vi "Begin.vi"(8 "error in":errorcluster) -> (0 "error out":errorcluster)   [LabVIEW 2020]
doc: "Called before other user functions, this VI is expected to open initial I/O refnums, load in file data, and do all program initialization. Notice that the <B>error out</B> terminal is simply used for data flow. Wiring it to other structures or subVIs ensures that this VI runs first."
uses:
  <vilib>/Rock Robotics/WPI/DriverStation/WPI_DriverStationRobotMode2.ctl
  <vilib>/Rock Robotics/WPI/ThirdParty/REV Robotics/REVLib/Typedef/Spark MAX Motor Type.ctl
  <vilib>/Rock Robotics/WPI/ThirdParty/REV Robotics/REVLib/Typedef/Spark MAX Sensor Type.ctl
  <vilib>/Rock Robotics/WPI/Joystick/WPI_JoystickDeviceEnum.ctl
  <vilib>/Rock Robotics/WPI/Solenoid/WPI_SolenoidChannel.ctl
  <vilib>/Rock Robotics/WPI/SafetyOutput/WPI_SafetyOutputConfigMenu.ctl
  <vilib>/Rock Robotics/SystemInterfaces/DIO/FPGA_DIOChannel.ctl
  Robot Global Data.vi
  <vilib>/Rock Robotics/Network Tables/NT Write String Array.vi
  <vilib>/Rock Robotics/WPI/RobotDrive/WPI_RobotDriveOpen2MotorWithExistingMotors.vi
  <vilib>/Rock Robotics/WPI/Solenoid/WPI_SolenoidOpenDouble.vi
  <vilib>/Rock Robotics/WPI/Utilities/WPI_GetSetVariantRefNum.vi
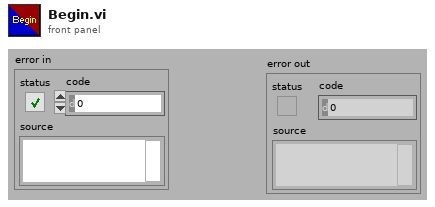
[diagram p1: front panel]
types:
  T1 = typedef "Spark MAX Sensor Type.ctl" = enum16{"No Sensor", "Hall Sensor", "Encoder", "-Not Available-", "Analog", "Alternate Encoder"}
  T2 = typedef "Spark MAX Motor Type.ctl" = enum16{"Brushed", "Brushless"}
  T3 = typedef "FPGA_DIOChannel.ctl" = enum8{"DIO 0", "DIO 1", "DIO 2", "DIO 3", "DIO 4", "DIO 5", "DIO 6", "DIO 7", "DIO 8", "DIO 9", "DIO MXP 0", "DIO MXP 1", "DIO MXP 2", "DIO MXP 3", "DIO MXP 4", "DIO MXP 5", "DIO MXP 6", "DIO MXP 7", "DIO MXP 8", "DIO MXP 9", "DIO MXP 10", "DIO MXP 11", "DIO MXP 12", "DIO MXP 13", "DIO MXP 14", "DIO MXP 15", "SPI Port CS1", "SPI Port CS2", "SPI Port CS3", "SPI Port MISO", "SPI Port MOSI", "Invalid"}
  T4 = typedef "WPI_SafetyOutputConfigMenu.ctl" = enum16{"Enable", "Disable"}
  T5 = typedef "WPI_SolenoidChannel.ctl" = enum8{"Solenoid 0", "Solenoid 1", "Solenoid 2", "Solenoid 3", "Solenoid 4", "Solenoid 5", "Solenoid 6", "Solenoid 7", "Solenoid 8", "Solenoid 9", "Solenoid 10", "Solenoid 11", "Solenoid 12", "Solenoid 13", "Solenoid 14", "Solenoid 15", "Invalid"}
  T6 = typedef "WPI_JoystickDeviceEnum.ctl" = enum16{"USB 0", "USB 1", "USB 2", "USB 3", "USB 4", "USB 5"}
  T7 = typedef "WPI_DriverStationRobotMode2.ctl" = enum16{"Autonomous Disabled", "Autonomous Enabled", "Teleop Disabled", "Teleop Enabled", "Disconnected", "Finish", "Test Disabled", "Test Enabled", "Emergency Stopped"}
  T8 = typedef "WPI_MotorControlDeviceRef.ctl" = cluster{"DeviceStatus":errorcluster, "Type":T9, "PWM":cluster{"PWM Channel":T10, "DeadBand":T11}, "CAN":cluster{"Device Number":u8, "SetOutput VI Ref":variant, "GetOutput VI Ref":variant, "Enable VI Ref":variant, "Disable VI Ref":variant, "Data":variant}, "Invert":bool, "DIO PWM":cluster{"PWM \"Enable\" Channel":T10, "DIOChannel":T3, "PWM Rate":dbl}}
  T9 = typedef "WPI_MotorControlType.ctl" = enum16{"PWM", "CAN", "DIO PWM"}
  T10 = typedef "FPGA_DIOPWMChannel.ctl" = enum8{"PWM 0", "PWM 1", "PWM 2", "PWM 3", "PWM 4", "PWM 5", "PWM 6", "PWM 7", "PWM 8", "PWM 9", "PWM MXP 0", "PWM MXP 1", "PWM MXP 2", "PWM MXP 3", "PWM MXP 4", "PWM MXP 5", "PWM MXP 6", "PWM MXP 7", "PWM MXP 8", "PWM MXP 9", "Invalid"}
  T11 = typedef "WPI_PWMDeadband.ctl" = cluster{"Name":string, "maxPositivePwm":i32, "minPositivePwm":i32, "centerPwm":i32, "maxNegativePwm":i32, "minNegativePwm":i32, "angularRange":u16}
  T12 = typedef "WPI_JoystickDevRef.ctl" = cluster{"Device":T6}
  T13 = typedef "WPI_RobotDriveDevRef.ctl" = cluster{"DevStatus":errorcluster, "Motors[]":T8[], "Square Inputs":bool, "Max Output":dbl}
  T14 = typedef "WPI_SolenoidDevRef.ctl" = cluster{"DevStatus":errorcluster, "Pneumatics Control Module":u8, "Forward Solenoid Channel":T5, "Reverse Solenoid Channel":T5}
  T15 = typedef "WPI_CompressorDevRef.ctl" = cluster{"DevStatus":errorcluster, "Pneumatics Control Module":u8}
  T16 = typedef "WPI_DigitalInputDevRef.ctl" = cluster{"DevStatus":errorcluster, "DIO Channel":T3}
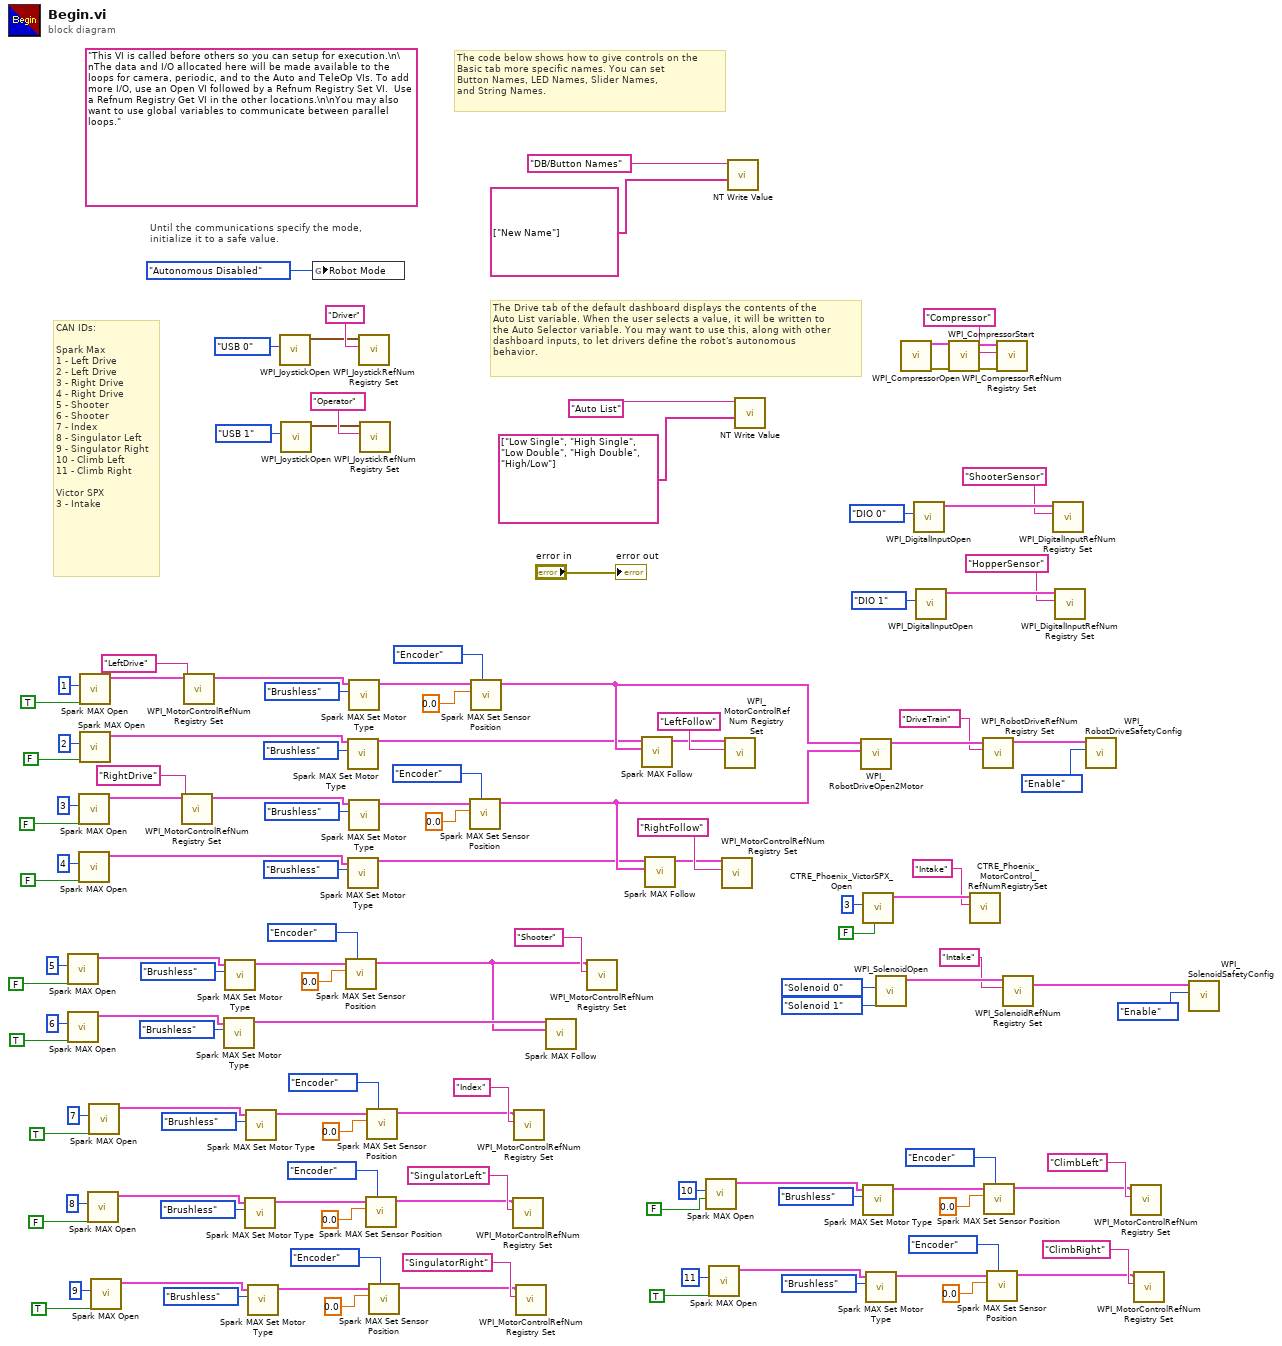
[diagram p0: block diagram]
diagram:
  (unwired) "This VI is called before others so you can setup for execution.\n\nThe data and I/O allocated here will be made available to the loops for camera, periodic, and to the Auto and TeleOp VIs. To add more I/O, use an Open VI followed by a Refnum Registry Set VI.  Use a Refnum Registry Get VI in the other locations.\n\nYou may also want to use global variables to communicate between parallel loops."
  # "CAN IDs:\n\nSpark Max\n1 - Left Drive\n2 - Left Drive\n3 - Right Drive\n4 - Right Drive\n5 - Shooter\n6 - Shooter\n7 - Index\n8 - Singulator Left\n9 - Singulator Right\n10 - Climb Left\n11 - Climb Right\n\nVictor SPX\n3 - Intake"
  # "The Drive tab of the default dashboard displays the contents of the\nAuto List variable. When the user selects a value, it will be written to\nthe Auto Selector variable. You may want to use this, along with other\ndashboard inputs, to let drivers define the robot's autonomous\nbehavior."
  # "The code below shows how to give controls on the\nBasic tab more specific names. You can set\nButton Names, LED Names, Slider Names,\nand String Names."
  # "Until the communications specify the mode,\ninitialize it to a safe value."
  n1 = call <vilib>:"Spark MAX Open.vi"("Invert"=FALSE, "Device Number"=u8 5) -> ("MotorControlDeviceRef"=w81:T8)  [unwired: 8 in, 1 out]
  n2 = call <vilib>:"Spark MAX Open.vi"("Invert"=TRUE, "Device Number"=u8 6) -> ("MotorControlDeviceRef"=w80:T8)  [unwired: 8 in, 1 out]
  n3 = call <vilib>:"Spark MAX Open.vi"("Invert"=FALSE, "Device Number"=u8 3) -> ("MotorControlDeviceRef"=w90:T8)  [unwired: 8 in, 1 out]
  n4 = call <vilib>:"Spark MAX Open.vi"("Invert"=FALSE, "Device Number"=u8 4) -> ("MotorControlDeviceRef"=w112:T8)  [unwired: 8 in, 1 out]
  n5 = call <vilib>:"Spark MAX Open.vi"("Invert"=TRUE, "Device Number"=u8 1) -> ("MotorControlDeviceRef"=w93:T8)  [unwired: 8 in, 1 out]
  n6 = call <vilib>:"Spark MAX Open.vi"("Invert"=FALSE, "Device Number"=u8 2) -> ("MotorControlDeviceRef"=w113:T8)  [unwired: 8 in, 1 out]
  n7 = call <vilib>:"Spark MAX Open.vi"("Invert"=FALSE, "Device Number"=u8 8) -> ("MotorControlDeviceRef"=w64:T8)  [unwired: 8 in, 1 out]
  n8 = call <vilib>:"Spark MAX Open.vi"("Invert"=TRUE, "Device Number"=u8 7) -> ("MotorControlDeviceRef"=w55:T8)  [unwired: 8 in, 1 out]
  n9 = call <vilib>:"Spark MAX Open.vi"("Invert"=TRUE, "Device Number"=u8 9) -> ("MotorControlDeviceRef"=w46:T8)  [unwired: 8 in, 1 out]
  n10 = call <vilib>:"WPI_MotorControlRefNum Registry Set.vi"("refnum name"="RightDrive", "MotorControlDevRef"=w90) -> ("MotorControlDevRef"=w88:T8)  [unwired: 8 in, 1 out]
  n11 = call <vilib>:"WPI_MotorControlRefNum Registry Set.vi"("refnum name"="LeftDrive", "MotorControlDevRef"=w93) -> ("MotorControlDevRef"=w91:T8)  [unwired: 8 in, 1 out]
  n12 = call <vilib>:"Spark MAX Set Motor Type.vi"("Motor Type"=Spark_MAX_Motor_Type."Brushless", "MotorControlDevRef"=w80) -> ("MotorControlDeviceRef"=w75:T8)  [unwired: 8 in, 1 out]
  n13 = call <vilib>:"Spark MAX Set Motor Type.vi"("Motor Type"=Spark_MAX_Motor_Type."Brushless", "MotorControlDevRef"=w81) -> ("MotorControlDeviceRef"=w78:T8)  [unwired: 8 in, 1 out]
  n14 = call <vilib>:"Spark MAX Set Motor Type.vi"("Motor Type"=Spark_MAX_Motor_Type."Brushless", "MotorControlDevRef"=w64) -> ("MotorControlDeviceRef"=w62:T8)  [unwired: 8 in, 1 out]
  n15 = call <vilib>:"Spark MAX Set Motor Type.vi"("Motor Type"=Spark_MAX_Motor_Type."Brushless", "MotorControlDevRef"=w55) -> ("MotorControlDeviceRef"=w53:T8)  [unwired: 8 in, 1 out]
  n16 = call <vilib>:"Spark MAX Set Motor Type.vi"("Motor Type"=Spark_MAX_Motor_Type."Brushless", "MotorControlDevRef"=w46) -> ("MotorControlDeviceRef"=w44:T8)  [unwired: 8 in, 1 out]
  n17 = call <vilib>:"WPI_JoystickOpen.vi"("JoystickDevice"=WPI_JoystickDeviceEnum."USB 0") -> ("JoystickDevRef"=w72:T12)  [unwired: 10 in]
  n18 = call <vilib>:"WPI_JoystickOpen.vi"("JoystickDevice"=WPI_JoystickDeviceEnum."USB 1") -> ("JoystickDevRef"=w69:T12)  [unwired: 10 in]
  n19 = global write "Robot Global Data.vi" "Robot Mode"(WPI_DriverStationRobotMode2."Autonomous Disabled" ("Robot Mode")) -> ()
  n20 = call <vilib>:"Spark MAX Set Sensor Position.vi"("Sensor Type (Hall Sensor)"=Spark_MAX_Sensor_Type."Encoder", "Position"=0.0, "MotorControlDeviceRef"=w78) -> ("MotorControlDeviceRef"=w74:T8)  [unwired: 7 in, 1 out]
  n21 = call <vilib>:"Spark MAX Set Motor Type.vi"("Motor Type"=Spark_MAX_Motor_Type."Brushless", "MotorControlDevRef"=w113) -> ("MotorControlDeviceRef"=w94:T8)  [unwired: 8 in, 1 out]
  n22 = call <vilib>:"Spark MAX Set Motor Type.vi"("Motor Type"=Spark_MAX_Motor_Type."Brushless", "MotorControlDevRef"=w112) -> ("MotorControlDeviceRef"=w97:T8)  [unwired: 8 in, 1 out]
  n23 = call <vilib>:"Spark MAX Set Motor Type.vi"("Motor Type"=Spark_MAX_Motor_Type."Brushless", "MotorControlDevRef"=w91) -> ("MotorControlDeviceRef"=w107:T8)  [unwired: 8 in, 1 out]
  n24 = call <vilib>:"Spark MAX Set Motor Type.vi"("Motor Type"=Spark_MAX_Motor_Type."Brushless", "MotorControlDevRef"=w88) -> ("MotorControlDeviceRef"=w108:T8)  [unwired: 8 in, 1 out]
  n25 = call <vilib>:"WPI_JoystickRefNum Registry Set.vi"("refnum name"="Driver", "JoystickDevRef"=w72) -> ()  [unwired: 8 in, 2 out]
  n26 = call <vilib>:"WPI_JoystickRefNum Registry Set.vi"("refnum name"="Operator", "JoystickDevRef"=w69) -> ()  [unwired: 8 in, 2 out]
  n27 = call <vilib>:"Spark MAX Set Sensor Position.vi"("Sensor Type (Hall Sensor)"=Spark_MAX_Sensor_Type."Encoder", "Position"=0.0, "MotorControlDeviceRef"=w62) -> ("MotorControlDeviceRef"=w59:T8)  [unwired: 7 in, 1 out]
  n28 = call <vilib>:"Spark MAX Set Sensor Position.vi"("Sensor Type (Hall Sensor)"=Spark_MAX_Sensor_Type."Encoder", "Position"=0.0, "MotorControlDeviceRef"=w53) -> ("MotorControlDeviceRef"=w50:T8)  [unwired: 7 in, 1 out]
  n29 = call <vilib>:"Spark MAX Set Sensor Position.vi"("Sensor Type (Hall Sensor)"=Spark_MAX_Sensor_Type."Encoder", "Position"=0.0, "MotorControlDeviceRef"=w44) -> ("MotorControlDeviceRef"=w41:T8)  [unwired: 7 in, 1 out]
  n30 = call <vilib>:"Spark MAX Set Sensor Position.vi"("Sensor Type (Hall Sensor)"=Spark_MAX_Sensor_Type."Encoder", "Position"=0.0, "MotorControlDeviceRef"=w108) -> ("MotorControlDeviceRef"=w98:T8)  [unwired: 7 in, 1 out]
  n31 = call <vilib>:"Spark MAX Set Sensor Position.vi"("Sensor Type (Hall Sensor)"=Spark_MAX_Sensor_Type."Encoder", "Position"=0.0, "MotorControlDeviceRef"=w107) -> ("MotorControlDeviceRef"=w95:T8)  [unwired: 7 in, 1 out]
  n32 = call <vilib>:"WPI_MotorControlRefNum Registry Set.vi"("refnum name"="SingulatorLeft", "MotorControlDevRef"=w59) -> ()  [unwired: 8 in, 2 out]
  n33 = call <vilib>:"WPI_MotorControlRefNum Registry Set.vi"("refnum name"="Index", "MotorControlDevRef"=w50) -> ()  [unwired: 8 in, 2 out]
  n34 = call <vilib>:"WPI_MotorControlRefNum Registry Set.vi"("refnum name"="SingulatorRight", "MotorControlDevRef"=w41) -> ()  [unwired: 8 in, 2 out]
  n35 = call <vilib>:"Spark MAX Follow.vi"("Master Controller"=w74, "MotorControlDeviceRef"=w75) -> ()  [unwired: 8 in, 2 out]
  n36 = call <vilib>:"WPI_MotorControlRefNum Registry Set.vi"("refnum name"="Shooter", "MotorControlDevRef"=w74) -> ()  [unwired: 8 in, 2 out]
  n37 = call <vilib>:"Spark MAX Follow.vi"("Master Controller"=w95, "MotorControlDeviceRef"=w94) -> ("MotorControlDeviceRef"=w96:T8)  [unwired: 8 in, 1 out]
  n38 = call <vilib>:"Spark MAX Follow.vi"("Master Controller"=w98, "MotorControlDeviceRef"=w97) -> ("MotorControlDeviceRef"=w99:T8)  [unwired: 8 in, 1 out]
  n39 = call <vilib>:"Spark MAX Open.vi"("Invert"=FALSE, "Device Number"=u8 10) -> ("MotorControlDeviceRef"=w15:T8)  [unwired: 8 in, 1 out]
  n40 = call <vilib>:"Spark MAX Open.vi"("Invert"=TRUE, "Device Number"=u8 11) -> ("MotorControlDeviceRef"=w6:T8)  [unwired: 8 in, 1 out]
  n41 = call <vilib>:"WPI_MotorControlRefNum Registry Set.vi"("refnum name"="RightFollow", "MotorControlDevRef"=w99) -> ()  [unwired: 8 in, 2 out]
  n42 = call <vilib>:"WPI_MotorControlRefNum Registry Set.vi"("refnum name"="LeftFollow", "MotorControlDevRef"=w96) -> ()  [unwired: 8 in, 2 out]
  n43 = call-poly <vilib>:"NT Write Value.vi"("String Array"=string[] ["New Name"], "Name"="DB/Button Names") -> ()  [unwired: 9 in, 1 out]
  n44 = call-poly <vilib>:"NT Write Value.vi"("String Array"=string[] ["Low Single", "High Single", "Low Double", "High Double", "High/Low"], "Name"="Auto List") -> ()  [unwired: 9 in, 1 out]
  n45 = call-poly <vilib>:"WPI_RobotDriveOpen2Motor.vi"("Right Motor Dev Ref"=w98, "Left Motor Dev Ref"=w95) -> ("RobotDriveDevRef"=w103:T13)  [unwired: 8 in, 1 out]
  n46 = call <vilib>:"CTRE_Phoenix_VictorSPX_Open.vi"("Invert"=FALSE, "Device Number"=u8 3) -> ("PhoenixMotorControlDevRef"=w39:T8)  [unwired: 8 in, 1 out]
  n47 = call <vilib>:"Spark MAX Set Motor Type.vi"("Motor Type"=Spark_MAX_Motor_Type."Brushless", "MotorControlDevRef"=w15) -> ("MotorControlDeviceRef"=w13:T8)  [unwired: 8 in, 1 out]
  n48 = call <vilib>:"Spark MAX Set Motor Type.vi"("Motor Type"=Spark_MAX_Motor_Type."Brushless", "MotorControlDevRef"=w6) -> ("MotorControlDeviceRef"=w4:T8)  [unwired: 8 in, 1 out]
  n49 = call-poly <vilib>:"WPI_SolenoidOpen.vi"("Reverse Solenoid Channel"=WPI_SolenoidChannel."Solenoid 1", "Forward Solenoid Channel"=WPI_SolenoidChannel."Solenoid 0") -> ("SolenoidDevRef"=w34:T14)  [unwired: 8 in, 1 out]
  n50 = call <vilib>:"WPI_CompressorOpen.vi"() -> ("CompressorDevRef"=w22:T15, "error out"=w23:errorcluster)  [unwired: 14 in]
  n51 = call <vilib>:"WPI_DigitalInputOpen.vi"("DIO Channel"=FPGA_DIOChannel."DIO 0") -> ("DigitalInputDevRef"=w28:T16)  [unwired: 9 in, 1 out]
  n52 = call <vilib>:"WPI_DigitalInputOpen.vi"("DIO Channel"=FPGA_DIOChannel."DIO 1") -> ("DigitalInputDevRef"=w25:T16)  [unwired: 9 in, 1 out]
  n53 = call <vilib>:"WPI_CompressorStart.vi"("error in (no error)"=w23, "CompressorDevRef"=w22) -> ("error out"=w21:errorcluster, "CompressorDevRef"=w20:T15)  [unwired: 8 in]
  n54 = call <vilib>:"CTRE_Phoenix_MotorControl_RefNumRegistrySet.vi"("refnum name"="Intake", "PhoenixMotorControlDevRef"=w39) -> ()  [unwired: 8 in, 2 out]
  n55 = call <vilib>:"WPI_RobotDriveRefNum Registry Set.vi"("refnum name"="DriveTrain", "RobotDriveDevRef"=w103) -> ("RobotDriveDevRef"=w101:T13)  [unwired: 8 in, 1 out]
  n56 = call <vilib>:"Spark MAX Set Sensor Position.vi"("Sensor Type (Hall Sensor)"=Spark_MAX_Sensor_Type."Encoder", "Position"=0.0, "MotorControlDeviceRef"=w13) -> ("MotorControlDeviceRef"=w10:T8)  [unwired: 7 in, 1 out]
  n57 = call <vilib>:"Spark MAX Set Sensor Position.vi"("Sensor Type (Hall Sensor)"=Spark_MAX_Sensor_Type."Encoder", "Position"=0.0, "MotorControlDeviceRef"=w4) -> ("MotorControlDeviceRef"=w1:T8)  [unwired: 7 in, 1 out]
  n58 = call <vilib>:"WPI_CompressorRefNum Registry Set.vi"("error in (no error)"=w21, "refnum name"="Compressor", "CompressorDevRef"=w20) -> ()  [unwired: 7 in, 2 out]
  n59 = call <vilib>:"WPI_SolenoidRefNum Registry Set.vi"("refnum name"="Intake", "SolenoidDevRef"=w34) -> ("SolenoidDevRef"=w32:T14)  [unwired: 8 in, 1 out]
  n60 = call <vilib>:"WPI_DigitalInputRefNum Registry Set.vi"("refnum name"="ShooterSensor", "DigitalInputDevRef"=w28) -> ()  [unwired: 8 in, 2 out]
  n61 = call <vilib>:"WPI_DigitalInputRefNum Registry Set.vi"("refnum name"="HopperSensor", "DigitalInputDevRef"=w25) -> ()  [unwired: 8 in, 2 out]
  n62 = call <vilib>:"WPI_RobotDriveSafetyConfig.vi"("mode"=WPI_SafetyOutputConfigMenu."Enable", "RobotDriveDevRef"=w101) -> ()  [unwired: 8 in, 2 out]
  n63 = call <vilib>:"WPI_MotorControlRefNum Registry Set.vi"("refnum name"="ClimbLeft", "MotorControlDevRef"=w10) -> ()  [unwired: 8 in, 2 out]
  n64 = call <vilib>:"WPI_MotorControlRefNum Registry Set.vi"("refnum name"="ClimbRight", "MotorControlDevRef"=w1) -> ()  [unwired: 8 in, 2 out]
  n65 = call <vilib>:"WPI_SolenoidSafetyConfig.vi"("mode"=WPI_SafetyOutputConfigMenu."Enable", "SolenoidDevRef"=w32) -> ()  [unwired: 8 in, 2 out]
  "error out" <- "error in"
